vi "Get All Points in ROI.vi"(8 "Error In":errorcluster, 11 "ROI Descriptor":T1 {"Contours"."Type" items=["No Selection", "Point", "Line", "Rectangle", "Oval", "Polygon", "Freehand Region", "Annulus", "Unused2", "Unused3", "Broken Line", "Freehand Line", "Rotated Rectangle"]}) -> (0 "Error Out":errorcluster, 3 "Point Array":cluster{"X":i32, "Y":i32}[](array[cluster]))   [LabVIEW 2021, in "Image.lvlib"]
uses:
  Image.lvlib
  <vilib>/vision/NI_Vision_Development_Module.lvlib
  Strings/Strings.lvlib
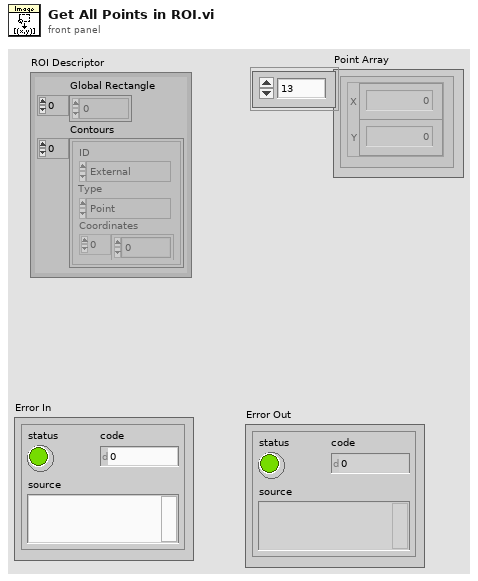
[diagram p1: front panel]
types:
  T1 = typedef "ROI Descriptor" = cluster{"Global Rectangle":i32[], "Contours":cluster{"ID":enum32{"External", "Internal"}, "Type":u32, "Coordinates":i32[]}[]}
  T2 = typedef "IMAQ Image.ctl" = refnum<image>
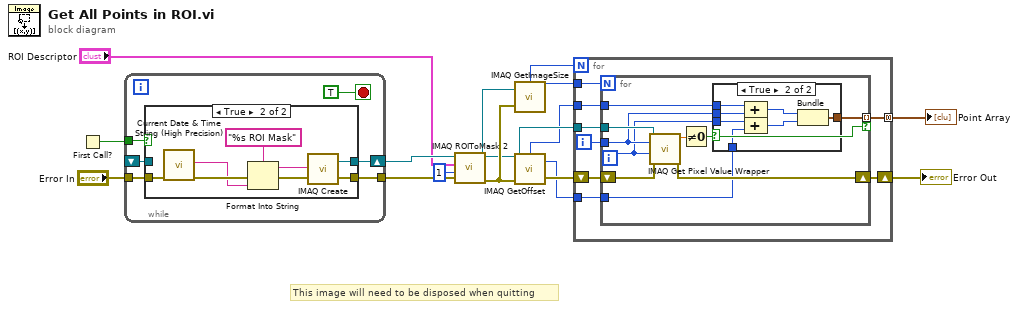
[diagram p0: block diagram]
diagram:
  # "This image will need to be disposed when quitting"
  n1 = First Call?() -> (First Call?: T/F=w15:bool)
  n2 = while {
    tunnel: w15 -> [w21]
    tunnel: "Error In" -> [w20]
    shift-right: [w19] -> w12
    shift-left: _ -> [w17]
    tunnel: [w16] -> w13
    stop <- TRUE stop-if-true
    n3 = case shown="True" w21 {
      tunnel: w20 -> [w22 w29]
      tunnel: [w23 w31] -> w19
      tunnel: w17 -> [w23 _]
      tunnel: [w22 w30] -> w16
      frame False {
      }
      frame True {
        n4 = call "Current Date & Time String (High Precision).vi"("Error In"=w29) -> ("Error Out"=w28:errorcluster, "time string"=w24:string)  [unwired: 7 in, 2 out]
        n5 = Format Into String(format string="%s ROI Mask" ("Image Name"), error in=w28, w24) -> (resulting string=w26:string, error out=w27:errorcluster)  [unwired: 1 in]
        n6 = call "IMAQ Create"("Image Name"=w26, "error in (no error)"=w27) -> ("New Image"=w31:T2, "error out"=w30:errorcluster)  [unwired: 3 in]
      }
    }
  }
  n7 = call "IMAQ ROIToMask 2"("error in (no error)"=w13, "Filling Value (255)"=1, "ROI Descriptor"="ROI Descriptor", "Image"=w12) -> ("error out"=w9:errorcluster, "Image Out"=w5:T2)  [unwired: 5 in, 1 out]
  n8 = call "IMAQ GetImageSize"("Image"=w5, "error in (no error)"=w9) -> ("Y Resolution"=w7:i32, "X Resolution"=w8:i32)  [unwired: 2 in, 1 out]
  n9 = call "IMAQ GetOffset"("Image"=w5, "error in (no error)"=w9) -> ("Y Offset"=w1:i32, "X Offset"=w2:i32, "error out"=w6:errorcluster)  [unwired: 2 in]
  n10 = for {
    N: w8 -> [_]
    tunnel: w7 -> [w39]
    shift-right: [w37] -> w3
    shift-left: w6 -> [w38]
    tunnel: w5 -> [w36]
    tunnel: [w34] -> w4 mode=concatenating
    tunnel: w2 -> [w33]
    tunnel: w1 -> [w32]
    i -> [w35]
    n11 = for {
      N: w39 -> [_]
      shift-right: [w47] -> w37
      shift-left: w38 -> [w48]
      tunnel: w36 -> [w49]
      tunnel: w35 -> [w45]
      tunnel: [w43] -> w34 mode=indexing if=w42
      tunnel: w33 -> [w41]
      tunnel: w32 -> [w40]
      i -> [w44]
      n12 = call "IMAQ Get Pixel Value Wrapper.vi"("Error In"=w48, "Y Coordinate"=w44, "X Coordinate"=w45, "Image"=w49) -> ("Error Out"=w47:errorcluster, "Pixel Value"=w46:sgl)  [unwired: 5 in, 1 out]
      n13 = Not Equal To 0?(x=w46) -> (x != 0?=w42:bool)
      n14 = case shown="True" w42 {
        tunnel: w45 -> [_ w56]
        tunnel: w44 -> [_ w55]
        tunnel: [_ w54] -> w43
        tunnel: w41 -> [_ w52]
        tunnel: w40 -> [_ w50]
        frame False {
        }
        frame True {
          n15 = Compound Arithmetic op=ADD(w52, w56) -> (w53:i32)
          n16 = Compound Arithmetic op=ADD(w55, w50) -> (w51:i32)
          n17 = Bundle(w53, w51) -> (w54:cluster{i32, i32})  [unwired: 1 in]
        }
      }
    }
  }
  "Error Out" <- w3
  "Point Array" <- w4
